vi "Stepper Speed (Set).vi"(6 "ISOBUS address":T4=-1 caption="ISOBUS address (-1)", 8 "error in":errorcluster, 9 "Unit":T1, 10 "Speed":u32 caption="Stepper Speed" max=7 step=1, 11 "Mercury Reference In":T5) -> (0 "error out":errorcluster, 2 "Response":T2, 3 "Mercury Reference Out":T5, 4 "Valid?":T3)   [LabVIEW 2014, in "Mercury iXX.lvlib" / "Auxiliary.lvlib"]
doc: "Set the current configuration for the Stepper speed setting."
uses:
  Auxiliary.lvlib
  Controls/Mercury Reference.ctl
  Controls/Comms Transport Layer.ctl
  Private/Controls/Query Dynamic Reference.ctl
  Controls/ISOBus Address.ctl
  Controls/Is Valid LED.ctl
  Controls/Response String.ctl
  Controls/Unit String.ctl
  Private/Controls/Command Verbs.ctl
  Mercury iXX.lvlib
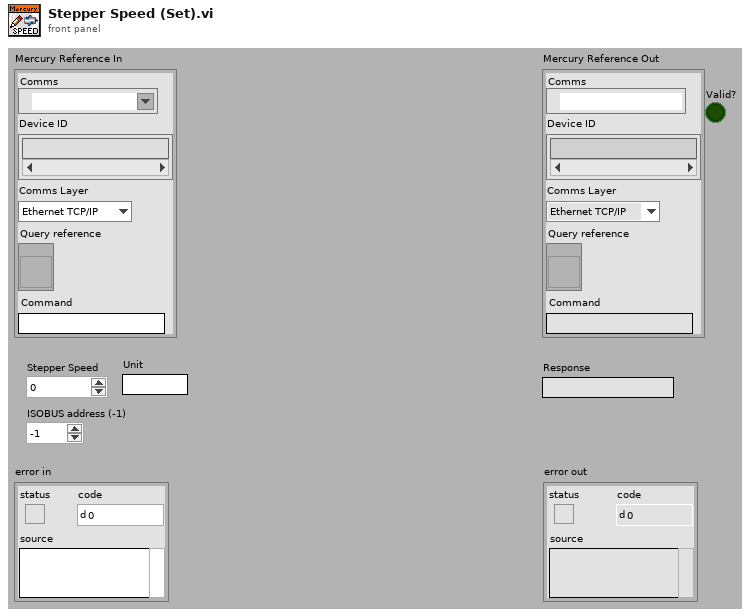
[diagram p1: front panel]
types:
  T1 = typedef "Mercury iXX.lvlib/Unit String.ctl" = string
  T2 = typedef "Mercury iXX.lvlib/Response String.ctl" = string
  T3 = typedef "Mercury iXX.lvlib/Is Valid LED.ctl" = bool
  T4 = typedef "Mercury iXX.lvlib/ISOBus Address.ctl" = i32
  T5 = typedef "Mercury iXX.lvlib/Mercury Reference.ctl" = cluster{"Comms":refnum<visa-resource-name>, "Device ID":string[], "Comms Layer":T6, "Command":string, "Query reference":T7}
  T6 = typedef "Mercury iXX.lvlib/Comms Transport Layer.ctl" = enum16{"Ethernet TCP/IP", "USB", "ISOBus - RS-232", "GPIB"}
  T7 = typedef "Mercury iXX.lvlib/Query Dynamic Reference.ctl" = refnum<vi>
  T8 = typedef "Mercury iXX.lvlib/Command Verbs.ctl" = string
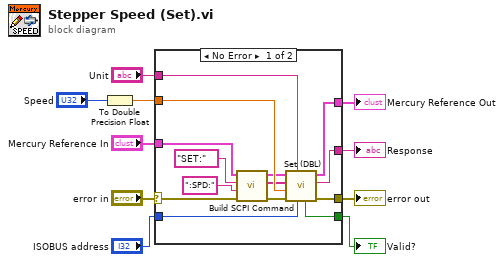
[diagram p0: block diagram]
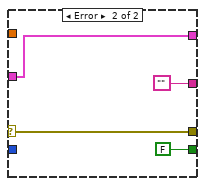
[diagram p2: hidden frame]
diagram:
  n1 = To Double Precision Float(number="Speed") -> (double precision float=w8:dbl)
  n2 = case shown="No Error" "error in" {
    selector: "error in" -> [w17 w27]
    tunnel: "Mercury Reference In" -> [w18 w28]
    tunnel: "ISOBUS address" -> [w24 _]
    tunnel: [w23 T3 FALSE ("Valid?")] -> w3
    tunnel: [w22 w27] -> w2
    tunnel: [w21 ""] -> w4
    tunnel: [w20 w28] -> w5
    tunnel: w8 -> [w19 _]
    tunnel: "Unit" -> [w11 _]
    frame No Error {
      n3 = call "Build SCPI Command.vi"("error in"=w17, "Noun(s)"=":SPD:" ("Command"), "Verb"=T8 "SET:", "Mercury Reference In"=w18) -> ("error out"=w14:errorcluster, "SCPI Message(s)"=w16:string[], "Mercury Reference Out"=w15:T5)  [unwired: 5 out]
      n4 = call "Set (DBL).vi"("ISOBUS address"=w24, "Unit"=w11, "error in"=w14, "Command Value (Dbl)"=w19, "SCPI Message(s)"=w16, "Mercury Reference In"=w15) -> ("error out"=w22:errorcluster, "Response"=w21:T2, "Mercury Reference Out"=w20:T5, "Valid?"=w23:T3)  [unwired: 2 out]
    }
    frame Error {
    }
  }
  "Mercury Reference Out" <- w5
  "error out" <- w2
  "Valid?" <- w3
  "Response" <- w4
